vi "Cluster Value.vi"(8 "error in (no error)":errorcluster, 9 "Enum Input":T1=enum."Startup", 10 "Vehicle Out of Position":bool, 11 "Data Car Wash":T2) -> (0 "error out":errorcluster, 3 "Data Car Wash Output":T2)   [LabVIEW 2021]
doc: "This VI manages the boolean value of the main cluster data in every state of the program to correctly update the indicators posteriorly."
uses:
  Controls/Car Wash Data.ctl
  Controls/Car Wash Indicators.ctl
  Controls/Wash Options.ctl
  Controls/Enum State Machine.ctl
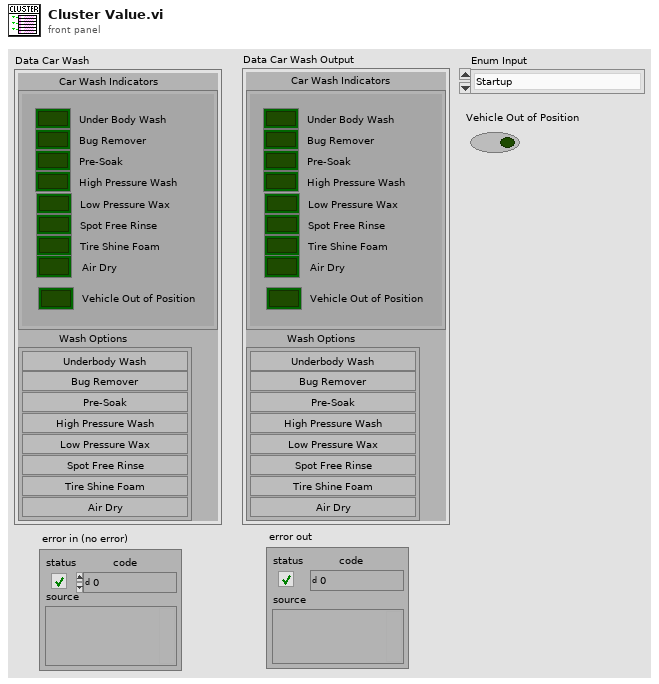
[diagram p1: front panel]
types:
  T1 = typedef "Enum State Machine.ctl" = enum16{"Entry", "Under Body Wash", "Bug Remover", "Pre-Soak", "High Pressure Wash", "Low Pressure Wax", "Spot Free Rinse", "Tire Shine Foam", "Air Dry", "Exit", "Startup", "Wait for Start", "Stop"}
  T2 = typedef "Car Wash Data.ctl" = cluster{"Car Wash Indicators":T3, "Wash Options":T4}
  T3 = typedef "Car Wash Indicators.ctl" = cluster{"Vehicle Out of Position":bool, "Under Body Wash":bool, "Bug Remover":bool, "Pre-Soak":bool, "High Pressure Wash":bool, "Low Pressure Wax":bool, "Spot Free Rinse":bool, "Tire Shine Foam":bool, "Air Dry":bool}
  T4 = typedef "Wash Options.ctl" = cluster{"Underbody Wash":bool, "Bug Remover":bool, "Pre-Soak":bool, "High Pressure Wash":bool, "Low Pressure Wax":bool, "Spot Free Rinse":bool, "Tire Shine Foam":bool, "Air Dry":bool}
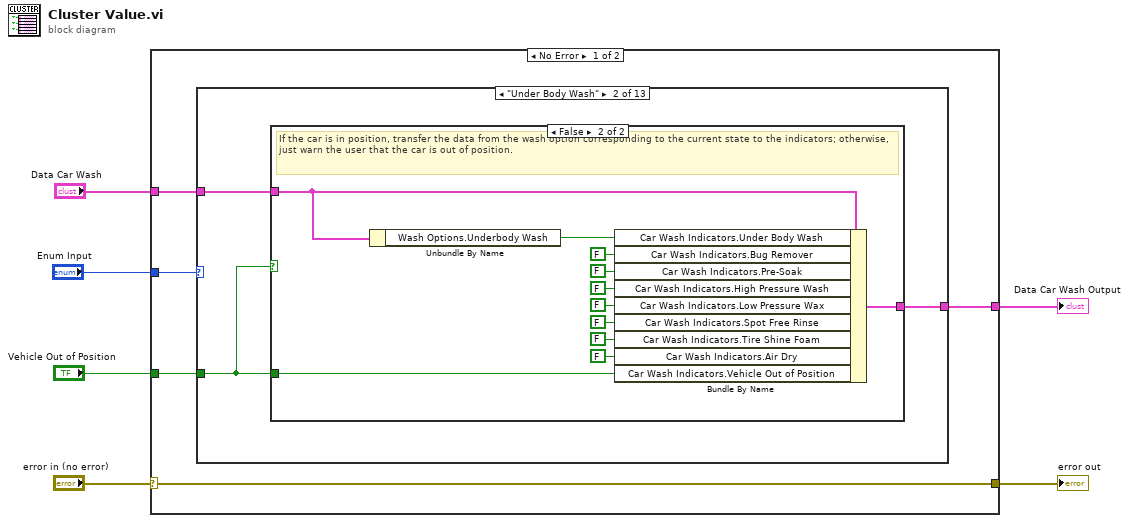
[diagram p0: block diagram]
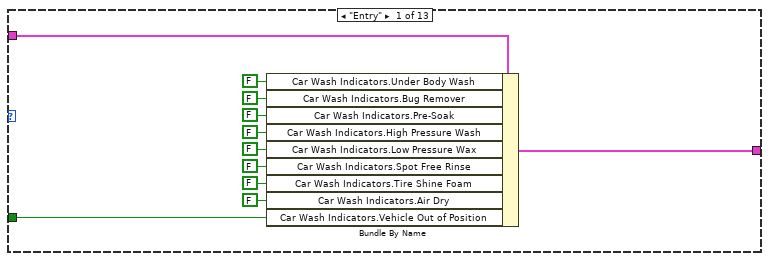
[diagram p2: hidden frame]
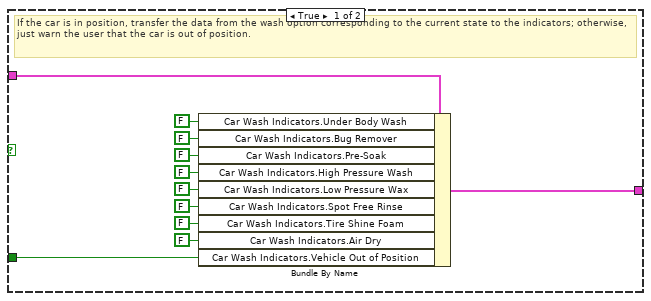
[diagram p3: hidden frame]
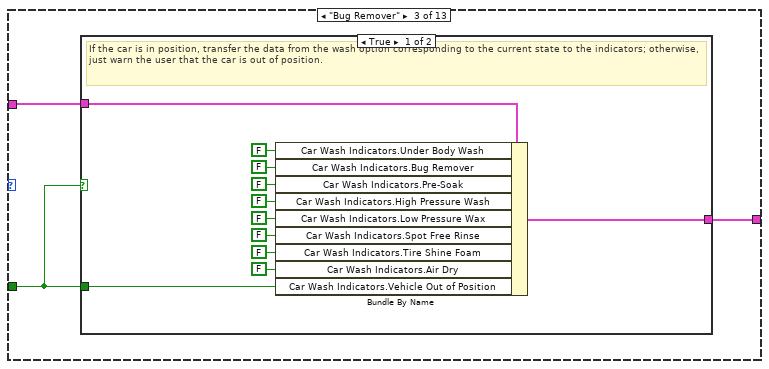
[diagram p4: hidden frame]
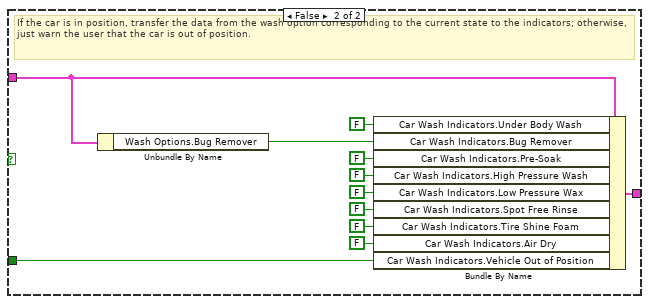
[diagram p5: hidden frame]
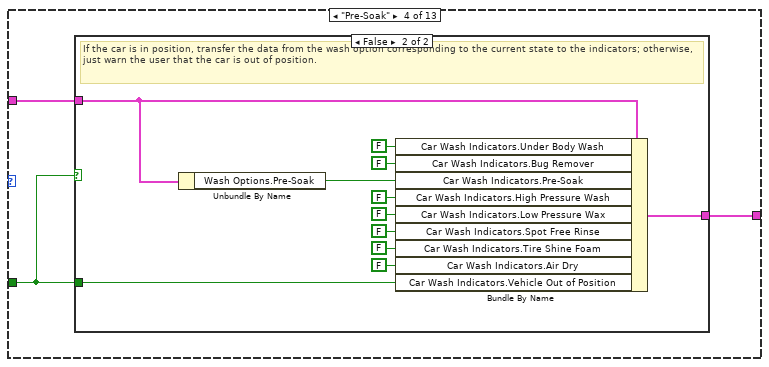
[diagram p6: hidden frame]
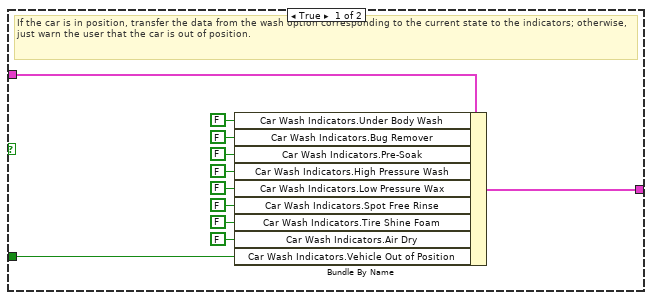
[diagram p7: hidden frame]
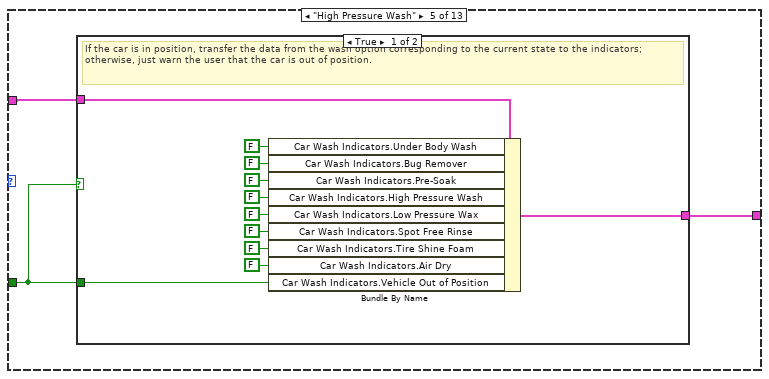
[diagram p8: hidden frame]
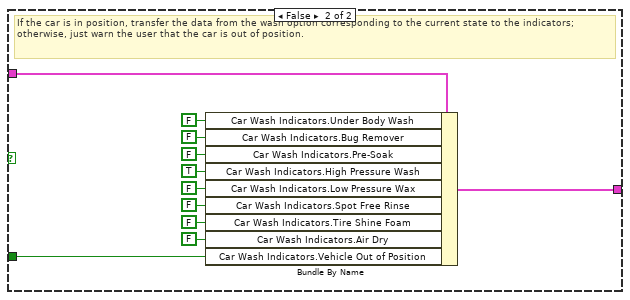
[diagram p9: hidden frame]
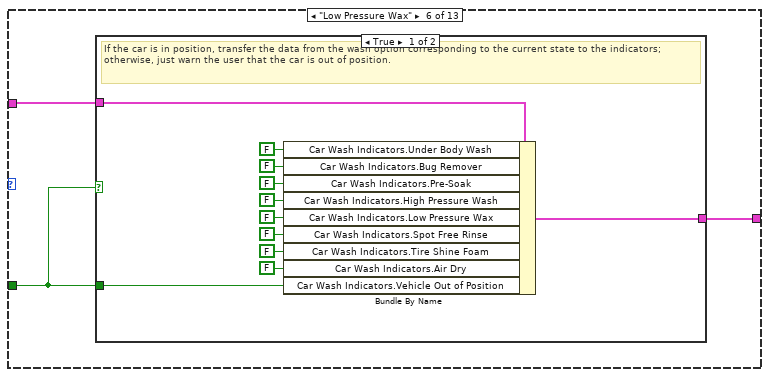
[diagram p10: hidden frame]
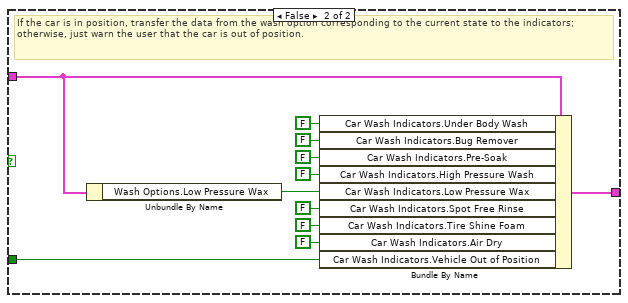
[diagram p11: hidden frame]
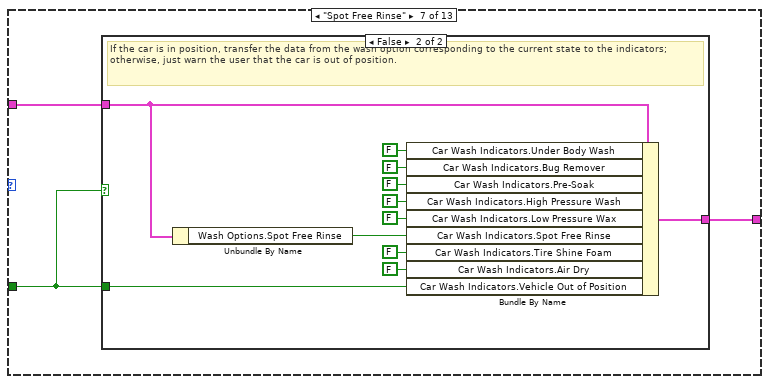
[diagram p12: hidden frame]
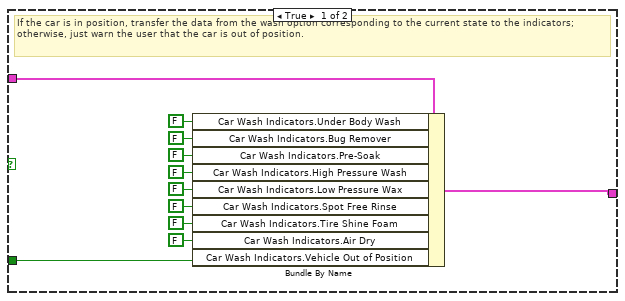
[diagram p13: hidden frame]
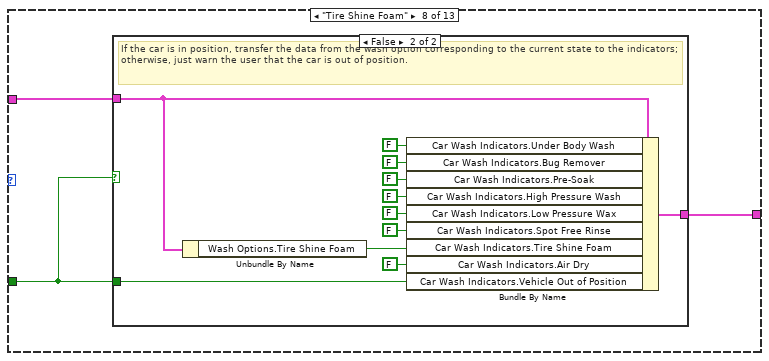
[diagram p14: hidden frame]
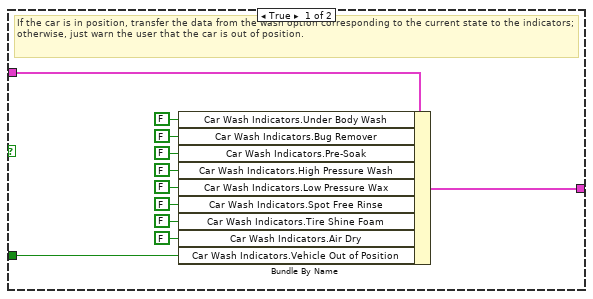
[diagram p15: hidden frame]
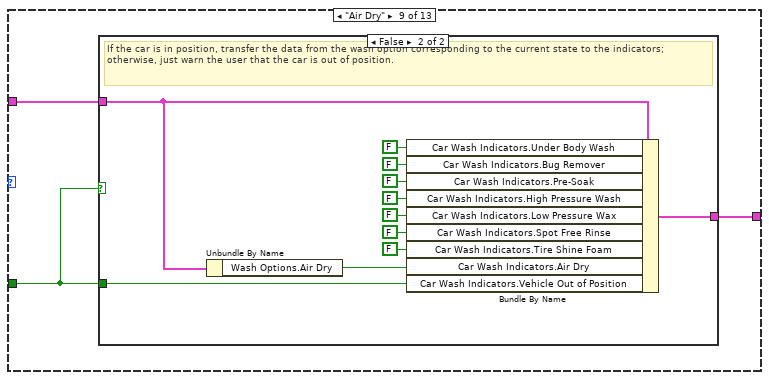
[diagram p16: hidden frame]
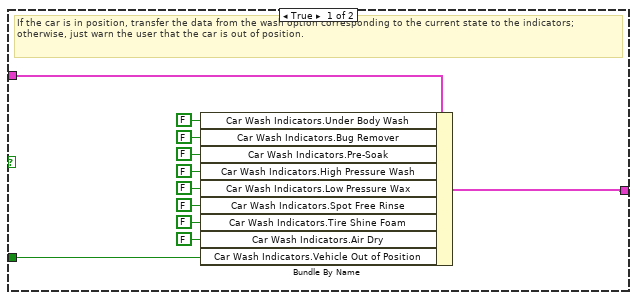
[diagram p17: hidden frame]
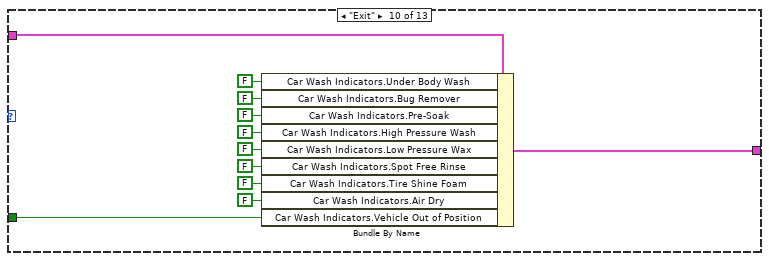
[diagram p18: hidden frame]
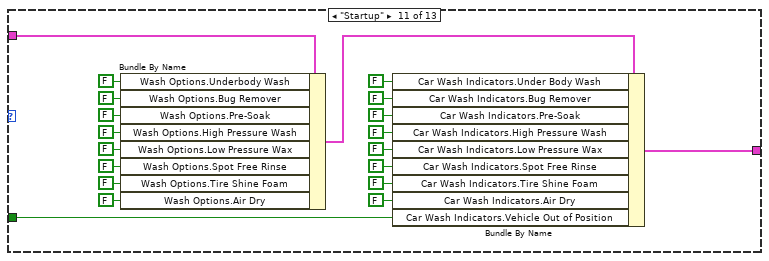
[diagram p19: hidden frame]
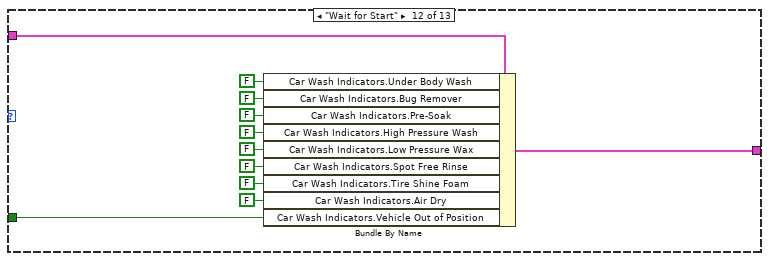
[diagram p20: hidden frame]
diagram:
  n1 = case shown="No Error" "error in (no error)" {
    selector: "error in (no error)" -> [w7 w277]
    tunnel: "Data Car Wash" -> [w11 w276]
    tunnel: [w10 w276] -> w5
    tunnel: "Vehicle Out of Position" -> [w9 _]
    tunnel: "Enum Input" -> [w8 _]
    tunnel: [w7 w277] -> w1
    frame No Error {
      n2 = case shown="\"Under Body Wash\"" w8 {
        tunnel: w11 -> [w14 w24 w49 w75 w100 w125 w150 w175 w200 w225 w244 w256 w266]
        tunnel: [w13 w25 w50 w74 w99 w124 w149 w174 w199 w224 w234 w255 w265] -> w10
        tunnel: w9 -> [w12 w23 w48 w73 w98 w123 w148 w173 w198 w223 w245 w254 w267]
        frame "Entry" {
          n3 = Bundle By Name(cluster=w14, "Car Wash Indicators.Under Body Wash"=FALSE, "Car Wash Indicators.Bug Remover"=FALSE, "Car Wash Indicators.Pre-Soak"=FALSE, "Car Wash Indicators.High Pressure Wash"=FALSE, "Car Wash Indicators.Low Pressure Wax"=FALSE, "Car Wash Indicators.Spot Free Rinse"=FALSE, "Car Wash Indicators.Tire Shine Foam"=FALSE, "Car Wash Indicators.Air Dry"=FALSE, "Car Wash Indicators.Vehicle Out of Position"=w12) -> (w13:T2)
        }
        frame "Under Body Wash" {
          n4 = case shown="False" w23 {
            tunnel: [w27 w40] -> w25
            tunnel: w24 -> [w28 w39]
            tunnel: w23 -> [w26 w38]
            frame True {
              # "If the car is in position, transfer the data from the wash option corresponding to the current state to the indicators; otherwise, just warn the user that the car is out of position."
              n5 = Bundle By Name(cluster=w28, "Car Wash Indicators.Under Body Wash"=FALSE, "Car Wash Indicators.Bug Remover"=FALSE, "Car Wash Indicators.Pre-Soak"=FALSE, "Car Wash Indicators.High Pressure Wash"=FALSE, "Car Wash Indicators.Low Pressure Wax"=FALSE, "Car Wash Indicators.Spot Free Rinse"=FALSE, "Car Wash Indicators.Tire Shine Foam"=FALSE, "Car Wash Indicators.Air Dry"=FALSE, "Car Wash Indicators.Vehicle Out of Position"=w26) -> (w27:T2)
            }
            frame False {
              # "If the car is in position, transfer the data from the wash option corresponding to the current state to the indicators; otherwise, just warn the user that the car is out of position."
              n6 = Unbundle By Name(w39) -> ("Wash Options.Underbody Wash"=w47:bool)
              n7 = Bundle By Name(cluster=w39, "Car Wash Indicators.Under Body Wash"=w47, "Car Wash Indicators.Bug Remover"=FALSE, "Car Wash Indicators.Pre-Soak"=FALSE, "Car Wash Indicators.High Pressure Wash"=FALSE, "Car Wash Indicators.Low Pressure Wax"=FALSE, "Car Wash Indicators.Spot Free Rinse"=FALSE, "Car Wash Indicators.Tire Shine Foam"=FALSE, "Car Wash Indicators.Air Dry"=FALSE, "Car Wash Indicators.Vehicle Out of Position"=w38) -> (w40:T2)
            }
          }
        }
        frame "Bug Remover" {
          n8 = case shown="True" w48 {
            tunnel: [w51 w65] -> w50
            tunnel: w49 -> [w53 w64]
            tunnel: w48 -> [w52 w63]
            frame True {
              # "If the car is in position, transfer the data from the wash option corresponding to the current state to the indicators; otherwise, just warn the user that the car is out of position."
              n9 = Bundle By Name(cluster=w53, "Car Wash Indicators.Under Body Wash"=FALSE, "Car Wash Indicators.Bug Remover"=FALSE, "Car Wash Indicators.Pre-Soak"=FALSE, "Car Wash Indicators.High Pressure Wash"=FALSE, "Car Wash Indicators.Low Pressure Wax"=FALSE, "Car Wash Indicators.Spot Free Rinse"=FALSE, "Car Wash Indicators.Tire Shine Foam"=FALSE, "Car Wash Indicators.Air Dry"=FALSE, "Car Wash Indicators.Vehicle Out of Position"=w52) -> (w51:T2)
            }
            frame False {
              # "If the car is in position, transfer the data from the wash option corresponding to the current state to the indicators; otherwise, just warn the user that the car is out of position."
              n10 = Unbundle By Name(w64) -> ("Wash Options.Bug Remover"=w72:bool)
              n11 = Bundle By Name(cluster=w64, "Car Wash Indicators.Under Body Wash"=FALSE, "Car Wash Indicators.Bug Remover"=w72, "Car Wash Indicators.Pre-Soak"=FALSE, "Car Wash Indicators.High Pressure Wash"=FALSE, "Car Wash Indicators.Low Pressure Wax"=FALSE, "Car Wash Indicators.Spot Free Rinse"=FALSE, "Car Wash Indicators.Tire Shine Foam"=FALSE, "Car Wash Indicators.Air Dry"=FALSE, "Car Wash Indicators.Vehicle Out of Position"=w63) -> (w65:T2)
            }
          }
        }
        frame "Pre-Soak" {
          n12 = case shown="False" w73 {
            tunnel: w75 -> [w77 w93]
            tunnel: [w76 w92] -> w74
            tunnel: w73 -> [w78 w91]
            frame True {
              # "If the car is in position, transfer the data from the wash option corresponding to the current state to the indicators; otherwise, just warn the user that the car is out of position."
              n13 = Bundle By Name(cluster=w77, "Car Wash Indicators.Under Body Wash"=FALSE, "Car Wash Indicators.Bug Remover"=FALSE, "Car Wash Indicators.Pre-Soak"=FALSE, "Car Wash Indicators.High Pressure Wash"=FALSE, "Car Wash Indicators.Low Pressure Wax"=FALSE, "Car Wash Indicators.Spot Free Rinse"=FALSE, "Car Wash Indicators.Tire Shine Foam"=FALSE, "Car Wash Indicators.Air Dry"=FALSE, "Car Wash Indicators.Vehicle Out of Position"=w78) -> (w76:T2)
            }
            frame False {
              # "If the car is in position, transfer the data from the wash option corresponding to the current state to the indicators; otherwise, just warn the user that the car is out of position."
              n14 = Unbundle By Name(w93) -> ("Wash Options.Pre-Soak"=w95:bool)
              n15 = Bundle By Name(cluster=w93, "Car Wash Indicators.Under Body Wash"=FALSE, "Car Wash Indicators.Bug Remover"=FALSE, "Car Wash Indicators.Pre-Soak"=w95, "Car Wash Indicators.High Pressure Wash"=FALSE, "Car Wash Indicators.Low Pressure Wax"=FALSE, "Car Wash Indicators.Spot Free Rinse"=FALSE, "Car Wash Indicators.Tire Shine Foam"=FALSE, "Car Wash Indicators.Air Dry"=FALSE, "Car Wash Indicators.Vehicle Out of Position"=w91) -> (w92:T2)
            }
          }
        }
        frame "High Pressure Wash" {
          n16 = case shown="True" w98 {
            tunnel: w100 -> [w102 w119]
            tunnel: [w103 w118] -> w99
            tunnel: w98 -> [w101 w117]
            frame True {
              # "If the car is in position, transfer the data from the wash option corresponding to the current state to the indicators; otherwise, just warn the user that the car is out of position."
              n17 = Bundle By Name(cluster=w102, "Car Wash Indicators.Under Body Wash"=FALSE, "Car Wash Indicators.Bug Remover"=FALSE, "Car Wash Indicators.Pre-Soak"=FALSE, "Car Wash Indicators.High Pressure Wash"=FALSE, "Car Wash Indicators.Low Pressure Wax"=FALSE, "Car Wash Indicators.Spot Free Rinse"=FALSE, "Car Wash Indicators.Tire Shine Foam"=FALSE, "Car Wash Indicators.Air Dry"=FALSE, "Car Wash Indicators.Vehicle Out of Position"=w101) -> (w103:T2)
            }
            frame False {
              # "If the car is in position, transfer the data from the wash option corresponding to the current state to the indicators; otherwise, just warn the user that the car is out of position."
              n18 = Bundle By Name(cluster=w119, "Car Wash Indicators.Under Body Wash"=FALSE, "Car Wash Indicators.Bug Remover"=FALSE, "Car Wash Indicators.Pre-Soak"=FALSE, "Car Wash Indicators.High Pressure Wash"=TRUE, "Car Wash Indicators.Low Pressure Wax"=FALSE, "Car Wash Indicators.Spot Free Rinse"=FALSE, "Car Wash Indicators.Tire Shine Foam"=FALSE, "Car Wash Indicators.Air Dry"=FALSE, "Car Wash Indicators.Vehicle Out of Position"=w117) -> (w118:T2)
            }
          }
        }
        frame "Low Pressure Wax" {
          n19 = case shown="True" w123 {
            tunnel: w125 -> [w127 w143]
            tunnel: [w128 w142] -> w124
            tunnel: w123 -> [w126 w141]
            frame True {
              # "If the car is in position, transfer the data from the wash option corresponding to the current state to the indicators; otherwise, just warn the user that the car is out of position."
              n20 = Bundle By Name(cluster=w127, "Car Wash Indicators.Under Body Wash"=FALSE, "Car Wash Indicators.Bug Remover"=FALSE, "Car Wash Indicators.Pre-Soak"=FALSE, "Car Wash Indicators.High Pressure Wash"=FALSE, "Car Wash Indicators.Low Pressure Wax"=FALSE, "Car Wash Indicators.Spot Free Rinse"=FALSE, "Car Wash Indicators.Tire Shine Foam"=FALSE, "Car Wash Indicators.Air Dry"=FALSE, "Car Wash Indicators.Vehicle Out of Position"=w126) -> (w128:T2)
            }
            frame False {
              # "If the car is in position, transfer the data from the wash option corresponding to the current state to the indicators; otherwise, just warn the user that the car is out of position."
              n21 = Unbundle By Name(w143) -> ("Wash Options.Low Pressure Wax"=w144:bool)
              n22 = Bundle By Name(cluster=w143, "Car Wash Indicators.Under Body Wash"=FALSE, "Car Wash Indicators.Bug Remover"=FALSE, "Car Wash Indicators.Pre-Soak"=FALSE, "Car Wash Indicators.High Pressure Wash"=FALSE, "Car Wash Indicators.Low Pressure Wax"=w144, "Car Wash Indicators.Spot Free Rinse"=FALSE, "Car Wash Indicators.Tire Shine Foam"=FALSE, "Car Wash Indicators.Air Dry"=FALSE, "Car Wash Indicators.Vehicle Out of Position"=w141) -> (w142:T2)
            }
          }
        }
        frame "Spot Free Rinse" {
          n23 = case shown="False" w148 {
            tunnel: w150 -> [w152 w168]
            tunnel: [w153 w167] -> w149
            tunnel: w148 -> [w151 w166]
            frame True {
              # "If the car is in position, transfer the data from the wash option corresponding to the current state to the indicators; otherwise, just warn the user that the car is out of position."
              n24 = Bundle By Name(cluster=w152, "Car Wash Indicators.Under Body Wash"=FALSE, "Car Wash Indicators.Bug Remover"=FALSE, "Car Wash Indicators.Pre-Soak"=FALSE, "Car Wash Indicators.High Pressure Wash"=FALSE, "Car Wash Indicators.Low Pressure Wax"=FALSE, "Car Wash Indicators.Spot Free Rinse"=FALSE, "Car Wash Indicators.Tire Shine Foam"=FALSE, "Car Wash Indicators.Air Dry"=FALSE, "Car Wash Indicators.Vehicle Out of Position"=w151) -> (w153:T2)
            }
            frame False {
              # "If the car is in position, transfer the data from the wash option corresponding to the current state to the indicators; otherwise, just warn the user that the car is out of position."
              n25 = Unbundle By Name(w168) -> ("Wash Options.Spot Free Rinse"=w169:bool)
              n26 = Bundle By Name(cluster=w168, "Car Wash Indicators.Under Body Wash"=FALSE, "Car Wash Indicators.Bug Remover"=FALSE, "Car Wash Indicators.Pre-Soak"=FALSE, "Car Wash Indicators.High Pressure Wash"=FALSE, "Car Wash Indicators.Low Pressure Wax"=FALSE, "Car Wash Indicators.Spot Free Rinse"=w169, "Car Wash Indicators.Tire Shine Foam"=FALSE, "Car Wash Indicators.Air Dry"=FALSE, "Car Wash Indicators.Vehicle Out of Position"=w166) -> (w167:T2)
            }
          }
        }
        frame "Tire Shine Foam" {
          n27 = case shown="False" w173 {
            tunnel: w175 -> [w178 w190]
            tunnel: [w177 w189] -> w174
            tunnel: w173 -> [w176 w188]
            frame True {
              # "If the car is in position, transfer the data from the wash option corresponding to the current state to the indicators; otherwise, just warn the user that the car is out of position."
              n28 = Bundle By Name(cluster=w178, "Car Wash Indicators.Under Body Wash"=FALSE, "Car Wash Indicators.Bug Remover"=FALSE, "Car Wash Indicators.Pre-Soak"=FALSE, "Car Wash Indicators.High Pressure Wash"=FALSE, "Car Wash Indicators.Low Pressure Wax"=FALSE, "Car Wash Indicators.Spot Free Rinse"=FALSE, "Car Wash Indicators.Tire Shine Foam"=FALSE, "Car Wash Indicators.Air Dry"=FALSE, "Car Wash Indicators.Vehicle Out of Position"=w176) -> (w177:T2)
            }
            frame False {
              # "If the car is in position, transfer the data from the wash option corresponding to the current state to the indicators; otherwise, just warn the user that the car is out of position."
              n29 = Unbundle By Name(w190) -> ("Wash Options.Tire Shine Foam"=w191:bool)
              n30 = Bundle By Name(cluster=w190, "Car Wash Indicators.Under Body Wash"=FALSE, "Car Wash Indicators.Bug Remover"=FALSE, "Car Wash Indicators.Pre-Soak"=FALSE, "Car Wash Indicators.High Pressure Wash"=FALSE, "Car Wash Indicators.Low Pressure Wax"=FALSE, "Car Wash Indicators.Spot Free Rinse"=FALSE, "Car Wash Indicators.Tire Shine Foam"=w191, "Car Wash Indicators.Air Dry"=FALSE, "Car Wash Indicators.Vehicle Out of Position"=w188) -> (w189:T2)
            }
          }
        }
        frame "Air Dry" {
          n31 = case shown="False" w198 {
            tunnel: w200 -> [w203 w215]
            tunnel: [w202 w214] -> w199
            tunnel: w198 -> [w201 w213]
            frame True {
              # "If the car is in position, transfer the data from the wash option corresponding to the current state to the indicators; otherwise, just warn the user that the car is out of position."
              n32 = Bundle By Name(cluster=w203, "Car Wash Indicators.Under Body Wash"=FALSE, "Car Wash Indicators.Bug Remover"=FALSE, "Car Wash Indicators.Pre-Soak"=FALSE, "Car Wash Indicators.High Pressure Wash"=FALSE, "Car Wash Indicators.Low Pressure Wax"=FALSE, "Car Wash Indicators.Spot Free Rinse"=FALSE, "Car Wash Indicators.Tire Shine Foam"=FALSE, "Car Wash Indicators.Air Dry"=FALSE, "Car Wash Indicators.Vehicle Out of Position"=w201) -> (w202:T2)
            }
            frame False {
              # "If the car is in position, transfer the data from the wash option corresponding to the current state to the indicators; otherwise, just warn the user that the car is out of position."
              n33 = Unbundle By Name(w215) -> ("Wash Options.Air Dry"=w216:bool)
              n34 = Bundle By Name(cluster=w215, "Car Wash Indicators.Under Body Wash"=FALSE, "Car Wash Indicators.Bug Remover"=FALSE, "Car Wash Indicators.Pre-Soak"=FALSE, "Car Wash Indicators.High Pressure Wash"=FALSE, "Car Wash Indicators.Low Pressure Wax"=FALSE, "Car Wash Indicators.Spot Free Rinse"=FALSE, "Car Wash Indicators.Tire Shine Foam"=FALSE, "Car Wash Indicators.Air Dry"=w216, "Car Wash Indicators.Vehicle Out of Position"=w213) -> (w214:T2)
            }
          }
        }
        frame "Exit" {
          n35 = Bundle By Name(cluster=w225, "Car Wash Indicators.Under Body Wash"=FALSE, "Car Wash Indicators.Bug Remover"=FALSE, "Car Wash Indicators.Pre-Soak"=FALSE, "Car Wash Indicators.High Pressure Wash"=FALSE, "Car Wash Indicators.Low Pressure Wax"=FALSE, "Car Wash Indicators.Spot Free Rinse"=FALSE, "Car Wash Indicators.Tire Shine Foam"=FALSE, "Car Wash Indicators.Air Dry"=FALSE, "Car Wash Indicators.Vehicle Out of Position"=w223) -> (w224:T2)
        }
        frame "Startup" {
          n36 = Bundle By Name(cluster=w244, "Wash Options.Underbody Wash"=FALSE, "Wash Options.Bug Remover"=FALSE, "Wash Options.Pre-Soak"=FALSE, "Wash Options.High Pressure Wash"=FALSE, "Wash Options.Low Pressure Wax"=FALSE, "Wash Options.Spot Free Rinse"=FALSE, "Wash Options.Tire Shine Foam"=FALSE, "Wash Options.Air Dry"=FALSE) -> (w235:T2)
          n37 = Bundle By Name(cluster=w235, "Car Wash Indicators.Under Body Wash"=FALSE, "Car Wash Indicators.Bug Remover"=FALSE, "Car Wash Indicators.Pre-Soak"=FALSE, "Car Wash Indicators.High Pressure Wash"=FALSE, "Car Wash Indicators.Low Pressure Wax"=FALSE, "Car Wash Indicators.Spot Free Rinse"=FALSE, "Car Wash Indicators.Tire Shine Foam"=FALSE, "Car Wash Indicators.Air Dry"=FALSE, "Car Wash Indicators.Vehicle Out of Position"=w245) -> (w234:T2)
        }
        frame "Wait for Start" {
          n38 = Bundle By Name(cluster=w256, "Car Wash Indicators.Under Body Wash"=FALSE, "Car Wash Indicators.Bug Remover"=FALSE, "Car Wash Indicators.Pre-Soak"=FALSE, "Car Wash Indicators.High Pressure Wash"=FALSE, "Car Wash Indicators.Low Pressure Wax"=FALSE, "Car Wash Indicators.Spot Free Rinse"=FALSE, "Car Wash Indicators.Tire Shine Foam"=FALSE, "Car Wash Indicators.Air Dry"=FALSE, "Car Wash Indicators.Vehicle Out of Position"=w254) -> (w255:T2)
        }
        frame "Stop" {
          n39 = Bundle By Name(cluster=w266, "Car Wash Indicators.Under Body Wash"=FALSE, "Car Wash Indicators.Bug Remover"=FALSE, "Car Wash Indicators.Pre-Soak"=FALSE, "Car Wash Indicators.High Pressure Wash"=FALSE, "Car Wash Indicators.Low Pressure Wax"=FALSE, "Car Wash Indicators.Spot Free Rinse"=FALSE, "Car Wash Indicators.Tire Shine Foam"=FALSE, "Car Wash Indicators.Air Dry"=FALSE, "Car Wash Indicators.Vehicle Out of Position"=w267) -> (w265:T2)
        }
      }
    }
    frame Error {
    }
  }
  "Data Car Wash Output" <- w5
  "error out" <- w1
